vi "Package Typed Message.vi"(8 "error in (no error)":errorcluster, 11 "StringGroup in":refnum<class "Group STR.lvclass">) -> (0 "error out":errorcluster, 2 "Data Msg":refnum<class "Message.lvclass">, 3 "StringGroup out":refnum<class "Group STR.lvclass">)   [LabVIEW 2020, in "Vecto.lvlib" / "Group STR.lvclass"]
uses:
  Group STR.lvclass
  Group STR.lvclass/Group STR.ctl
  Group/Group.lvclass
  Group Config/Group Config.lvclass
  lv-volatus/messages/StringData/Data.ctl
  lv-volatus/messages/StringData/StringData.lvlib
  lv-volatus/messages/StringData/Class/Msg.lvclass
  lv-protoc/LV-Proto/Message/Message.lvclass
  Vecto.lvlib
  C:/dev/lv20CE/relink/lv-vecto/Vecto/Group/Group.lvclass
  C:/dev/lv20CE/relink/lv-vecto/Vecto/Group STR/Group STR.lvclass
  C:/dev/lv20CE/relink/lv-volatus/messages/StringData/Class/Msg.lvclass
  C:/dev/lv20CE/relink/lv-protoc/LV-Proto/Message/Message.lvclass
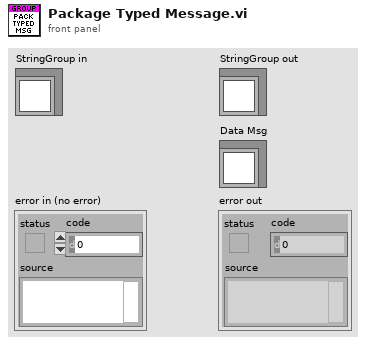
[diagram p1: front panel]
types:
  T1 = typedef "StringData.lvlib/Data.ctl" = cluster{"group_name":string, "data_timestamp":i64, "strings":string[], "names_crc":u32}
  T2 = typedef "Vecto.lvlib/StringGroup.lvclass/Ref.ctl" = cluster{"Strings":string[], "Timestamp":dbl[]}
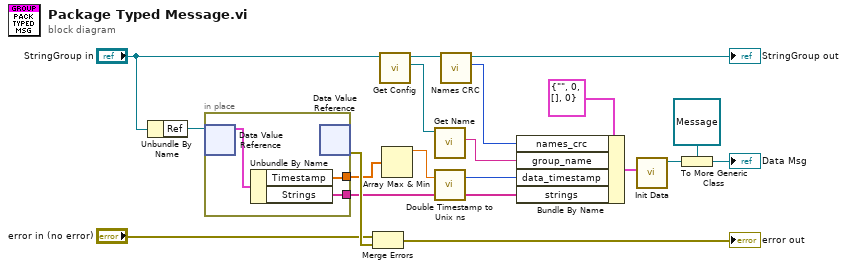
[diagram p0: block diagram]
diagram:
  n1 = Unbundle By Name("StringGroup in") -> ("Ref"=w17:refnum<data-value>)
  n2 = in-place {
    in-place-border: [w21] -> w8
    in-place-border: [w20] -> w15
    n3 = in-place-dvr #1(w17) -> (w22:T2)  [unwired: 1 out]
    n4 = Unbundle By Name(w22) -> ("Timestamp"=w20:dbl[], "Strings"=w21:string[])
    n5 = in-place-dvr #1() -> (w19:errorcluster)  [unwired: 1 in, 1 out]
  }
  n6 = Merge Errors("error in (no error)", w19) -> (→"error out":errorcluster)
  n7 = call "Get Config.vi"("Group in"="StringGroup in") -> ("Config"=w13:refnum<class "Group Config.lvclass">, "Group out"=w14:refnum<class "Group STR.lvclass">)  [unwired: 8 in, 1 out]
  n8 = Array Max & Min(array=w15) -> (max value=w9:dbl)  [unwired: 3 out]
  n9 = call "Get Name.vi"("Group Config in"=w13) -> ("Name"=w10:string)  [unwired: 8 in, 2 out]
  n10 = call "Double Timestamp to Unix ns.vi"("Timestamp"=w9) -> ("unix ns"=w11:i64)  [unwired: 2 in]
  n11 = call "Names CRC.vi"("Group in"=w14) -> ("Names CRC"=w1:u32, "Group out"=→"StringGroup out":refnum<class "Group STR.lvclass">)  [unwired: 9 in]
  n12 = Bundle By Name(cluster=T1 {"group_name"="", "data_timestamp"=0, "strings"=[], "names_crc"=0} ("StringData"), "names_crc"=w1, "group_name"=w10, "data_timestamp"=w11, "strings"=w8) -> (w7:T1)
  n13 = call "Init Data.vi"("Data"=w7) -> ("Msg out"=w5:refnum<class "Msg.lvclass">)  [unwired: 10 in]
  n14 = To More Generic Class(target class=refnum<class "Message.lvclass"> refnum ("LV-Proto.lvlib:Message.lvclass"), reference=w5) -> (generic class reference=→"Data Msg":refnum<class "Message.lvclass">)
